vi "AddDependency.vi"(7 "Level":string, 8 "error in (no error)":errorcluster, 10 "Dependency":refnum<class "SMO.lvclass">, 11 "SMO in":refnum<class "SMO.lvclass">) -> (0 "error out":errorcluster, 3 "SMO out":refnum<class "SMO.lvclass">)   [LabVIEW 2019, in "SMO.lvclass"]
doc: "JKI State Machine Objects (SMO) 1.3.0.56\nJKI - JKI\nCopyright (c) 2017, JKI"
uses:
  SMO.lvclass
  Typedefs/SMO Dependency--Cluster.ctl
  Typedefs/SMO Dependency Event--Cluster.ctl
  Typedefs/SMO Dependency Event--Enum.ctl
  SMO.lvclass/SMO.ctl
  <vilib>/regexp/Match Regular Expression.xnode
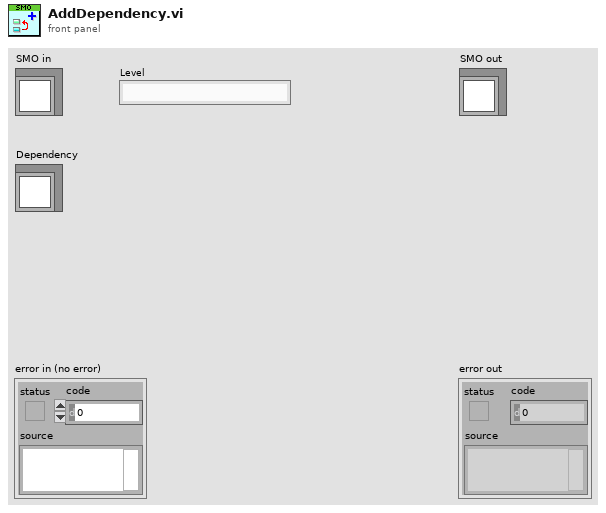
[diagram p1: front panel]
types:
  T1 = typedef "SMO.lvclass/SMO Dependency Event--Enum.ctl" = enum16{"Added", "Removed", "Started", "Stopped"}
  T2 = typedef "SMO.lvclass/SMO Dependency Event--Cluster.ctl" = cluster{"Name":string, "GUID":string, "Event":T1}
  T3 = typedef "SMO.lvclass/SMO Dependency--Cluster.ctl" = cluster{"Dependency":refnum<class "SMO.lvclass">, "Level":string}
  T4 = typedef "SMO.lvclass/PrivateData--Ref.ctl" = refnum<data-value>
  T5 = typedef "SMO.lvclass/PrivateData--Cluster.ctl" = cluster{"Parent Call":T6, "Registered Processes":T7[], "Sync Notifier":refnum<notifier>, "Process Error Notifier":refnum<notifier>, "Protected Events":T8, "Public Events":T9, "SMO State":T10, "[Dependencies]":T3[], "[Attributes]":refnum<class "Attribute.lvclass">[], "Launcher Close":refnum<notifier>, "Caller Watchdog":refnum<queue>, "Accessibility":T11, "NbStaticDependencies":u32}
  T6 = typedef "SMO.lvclass/Parent Call--Enum.ctl" = enum16{"Allows parent to run", "Does not request parent to run"}
  T7 = typedef "SMO.lvclass/RegisteredProcessData--Cluster.ctl" = cluster{"Name":string, "Static VI Ref":refnum<vi>, "Running":bool, "NotifierRef":u32}
  T8 = typedef "SMO.lvclass/Protected Events.ctl" = cluster{"StopProcesses":refnum<user-event>, "AbortProcesses":refnum<user-event>, "Config Changed":refnum<user-event>, "Dependency":refnum<user-event>}
  T9 = typedef "SMO.lvclass/Public Events.ctl" = cluster{"Error":refnum<user-event>, "State":refnum<user-event>, "Reserve State":refnum<user-event>}
  T10 = typedef "SMO.lvclass/SMOState --Enum.ctl" = enum16{"unknown", "Created", "Started", "Stopped"}
  T11 = typedef "SMO.lvclass/Accessibility--Cluster.ctl" = cluster{"Lock Key":string, "Reserve State":T12}
  T12 = typedef "SMO.lvclass/Reserve State--Enum.ctl" = enum16{"Unreserved", "Reserved", "Self-locked"}
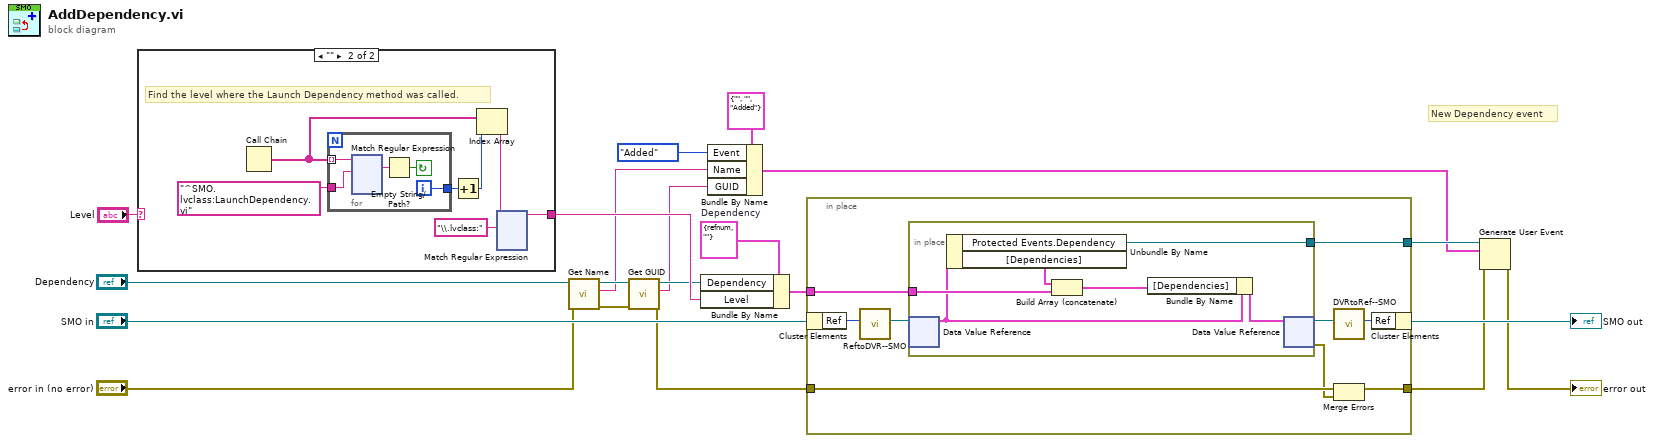
[diagram p0: block diagram]
diagram:
  w19 = T3 {"Dependency"=refnum, "Level"=""}  # Dependency
  # "New Dependency event"
  n1 = case shown="\"\"" "Level" {
    selector: "Level" -> [w21 _]
    tunnel: [w21 w22] -> w17
    frame Default {
    }
    frame "" {
      # "Find the level where the Launch Dependency method was called."
      n2 = Call Chain() -> (call chain=w27:string[])
      n3 = for {
        tunnel: w27 -> [w147] mode=indexing
        tunnel: "^SMO.lvclass:LaunchDependency.vi" -> [w146]
        tunnel: [w143] -> w26
        i -> [w143]
        stop <- w144 continue-if-true
        n4 = xnode "Match Regular Expression"("input string"=w147, "regular expression"=w146) -> ("whole match"=w145:string)  [unwired: 4 in, 4 out]
        n5 = Empty String/Path?(string/path=w145) -> (empty?=w144:bool)
      }
      n6 = Increment(x=w26) -> (x+1=w25:i32)
      n7 = Index Array(array=w27, index=w25) -> (element=w24:string)
      n8 = xnode "Match Regular Expression"("input string"=w24, "regular expression"="\\.lvclass:") -> ("before match"=w22:string)  [unwired: 4 in, 4 out]
    }
  }
  n9 = call "Get Name.vi"("error in (no error)"="error in (no error)", "SMO"="Dependency") -> ("error out"=w9:errorcluster, "Name"=w4:string, "SMO out"=w11:refnum<class "SMO.lvclass">)  [unwired: 7 in]
  n10 = call "Get GUID.vi"("error in (no error)"=w9, "SMO"=w11) -> ("error out"=w6:errorcluster, "GUID"=w3:string, "SMO out"=w10:refnum<class "SMO.lvclass">)  [unwired: 7 in]
  n11 = Bundle By Name(cluster=w19, "Dependency"=w10, "Level"=w17) -> (w18:T3)
  n12 = Bundle By Name(cluster=T2 {"Name"="", "GUID"="", "Event"=enum."Added"} ("Dependency Event"), "Event"=SMO_Dependency_Event--Enum."Added", "Name"=w4, "GUID"=w3) -> (w2:T2)
  n13 = in-place {
    in-place-border: w6 -> [w266]
    in-place-border: [w264] -> w13
    in-place-border: w18 -> [w263]
    in-place-border: [w262] -> w15
    n14 = in-place-cluster #1("SMO in") -> ("Ref"=w270:u32)
    n15 = call "ReftoDVR--SMO.vi"("Ref"=w270) -> ("Ref"=w269:T4)  [unwired: 10 in]
    n16 = in-place {
      in-place-border: w263 -> [w274]
      in-place-border: [w271] -> w262
      n17 = in-place-dvr #2(w269) -> (w272:T5)  [unwired: 1 out]
      n18 = Unbundle By Name(w272) -> ("Protected Events.Dependency"=w271:refnum<user-event>, "[Dependencies]"=w275:T3[])
      n19 = Build Array (concatenate)(w275, w274) -> (w273:T3[])
      n20 = Bundle By Name(cluster=w272, "[Dependencies]"=w273) -> (w276:T5)
      n21 = in-place-dvr #2(w276) -> (w268:T4, w265:errorcluster)
    }
    n22 = call "DVRtoRef--SMO.vi"("Ref"=w268) -> ("Ref"=w267:u32)  [unwired: 10 in]
    n23 = Merge Errors(w266, w265) -> (w264:errorcluster)
    n24 = in-place-cluster #1("Ref"=w267) -> (→"SMO out":refnum<class "SMO.lvclass">)
  }
  n25 = Generate User Event(user event=w15, event data cluster=w2, error in=w13) -> (error out=→"error out":errorcluster)  [unwired: 1 in, 1 out]
